vi "Dispose.vi"(8 "Error In":errorcluster, 11 "reference in":refnum<class "Wolfram.lvclass">) -> (0 "Error Out":errorcluster, 3 "reference out":refnum<class "Wolfram.lvclass">)   [LabVIEW 2020, in "Wolfram.lvclass"]
uses:
  Wolfram.lvclass
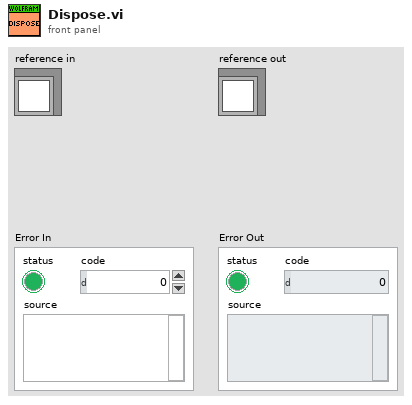
[diagram p1: front panel]
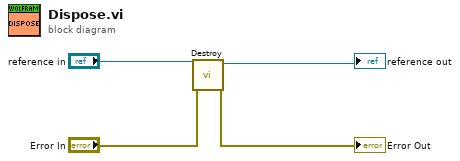
[diagram p0: block diagram]
diagram:
  n1 = call-dynamic "Destroy.vi"("error in (no error)"="Error In", "reference in"="reference in") -> ("error out"=→"Error Out":errorcluster, "reference out"=→"reference out":refnum<class "Wolfram.lvclass">)  [unwired: 8 in]
